vi "pulse_distribute_tester.vi"() -> ()   [LabVIEW 2021]
uses:
  <instrlib>/_niInstr/DSP/v1/Shared/Public/IQ Data.ctl
  pdw.ctl
  mode_type.ctl
  <instrlib>/_niInstr/Basic Elements/v1/FPGA/Private/Count Up U64.vi
  <instrlib>/_niInstr/Basic Elements/v1/FPGA/niInstr Basic Elements v1 FPGA.lvlib
  <instrlib>/_niInstr/DSP/v1/Shared/niInstr DSP v1 Shared.lvlib
panel:
  out "pulses read":u64=36
  out "free dds 4":bool=TRUE
  out "free dds 3":bool
  out "free dds 2":bool
  out "free dds":bool
  out "Boolean 4":bool
  out "Boolean 3":bool
  out "Boolean 2":bool
  out "Boolean":bool
  out "time":u64=655
  in  "stop":bool
  out "new pulse":bool
  out "free DDS":bool[](array[boolean])=[FALSE, FALSE, FALSE, TRUE]
  out "output cluster":T1 {"I" format="%#_6f"}
  out "get new poulse":bool=TRUE
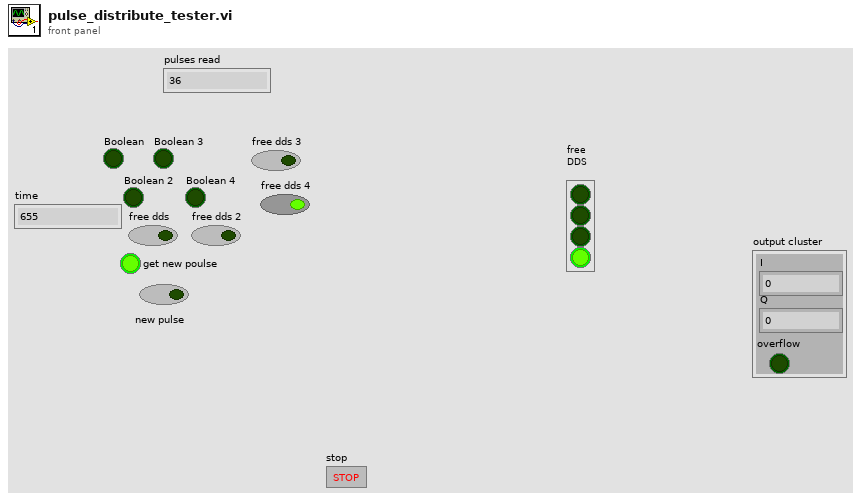
[diagram p1: front panel]
types:
  T1 = typedef "niInstr DSP v1 Shared.lvlib/IQ Data.ctl" = cluster{"I":fxp<+/-,18,1>, "Q":fxp<+/-,18,1>, "overflow":bool}
  T2 = typedef "pdw.ctl" = cluster{"PW":u32, "frequency shift":fxp<+/-,48,0>, "amp":fxp<+/-,18,1>, "mode type":T3, "mode depth":u32, "mode filter":u8, "phase shift":fxp<+/-,16,1>, "pulse shape filter":u8}
  T3 = typedef "mode_type.ctl" = enum8{"CW", "NC - CW", "NC - cw", "LFM", "BPSK", "QPSK"}
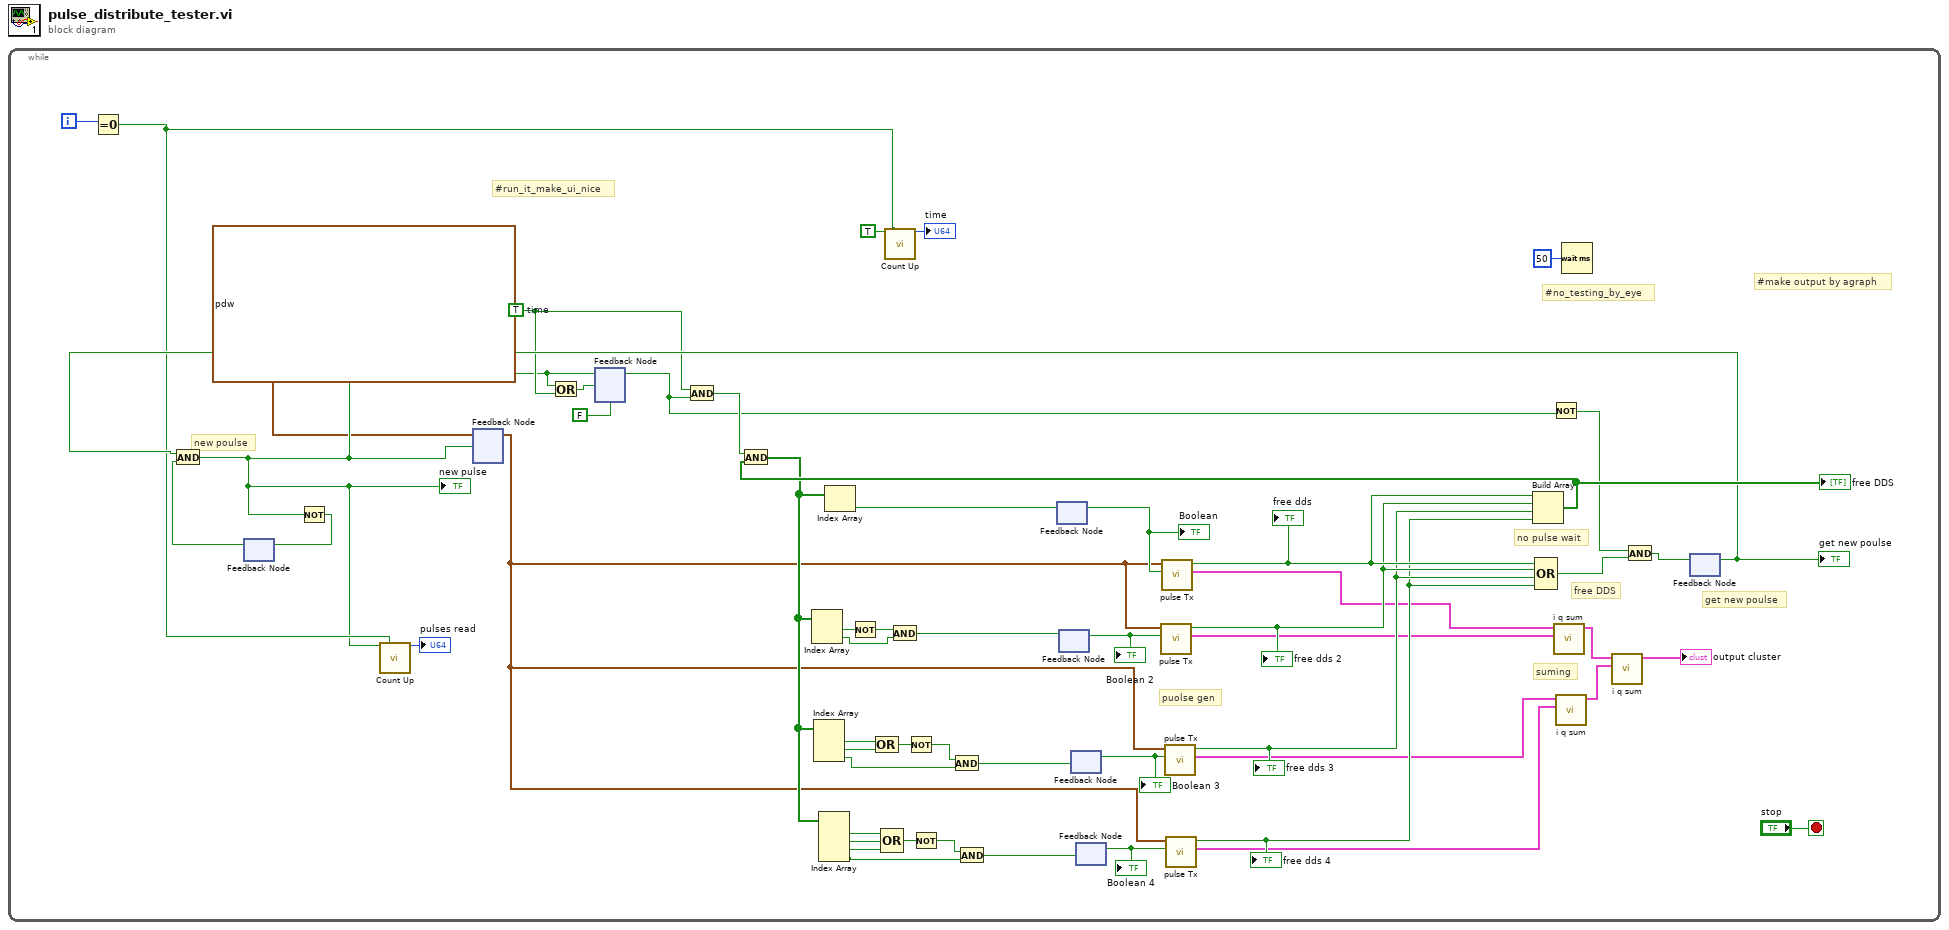
[diagram p0: block diagram]
diagram:
  n1 = while {
    i -> [w9]
    stop <- "stop" stop-if-true
    w5 = TRUE  # time
    # "#no_testing_by_eye"
    # "#make output by agraph"
    # "#run_it_make_ui_nice"
    # "new poulse"
    # "suming"
    # "puolse gen"
    # "get new poulse"
    # "no pulse wait"
    # "free DDS"
    n2 = Equal To 0?(x=w9) -> (x = 0?=w8:bool)
    n3 = feedback #1() -> (w11:bool)  [unwired: 1 in]
    n4 = feedback #2() -> (w1:T2)  [unwired: 1 in]
    n5 = feedback #3(FALSE ("Output Valid")) -> (w3:bool)
    n6 = And(x=w5, y=w3) -> (x .and. y?=w35:bool)
    n7 = call-poly <instrlib>:"Count Up.vi"("increment"=TRUE, "reset"=w8) -> ("count out"=→"time":u64)  [unwired: 13 in]
    n8 = feedback #4() -> (w23:bool)  [unwired: 1 in]
    "Boolean" <- w23
    n9 = feedback #5() -> (w46:bool)  [unwired: 1 in]
    "Boolean 2" <- w46
    n10 = feedback #6() -> (w45:bool)  [unwired: 1 in]
    "Boolean 3" <- w45
    n11 = feedback #7() -> (w43:bool)  [unwired: 1 in]
    "Boolean 4" <- w43
    n12 = call "pulse Tx.vi"("take it!"=w46, "Cluster"=w1) -> ("data out"=w29:T1, "free dds"=w55:bool)  [unwired: 5 in, 3 out]
    "free dds 2" <- w55
    n13 = call "pulse Tx.vi"("take it!"=w23, "Cluster"=w1) -> ("data out"=w30:T1, "free dds"=w56:bool)  [unwired: 5 in, 3 out]
    "free dds" <- w56
    n14 = call "pulse Tx.vi"("take it!"=w45, "Cluster"=w1) -> ("data out"=w28:T1, "free dds"=w44:bool)  [unwired: 5 in, 3 out]
    "free dds 3" <- w44
    n15 = call "pulse Tx.vi"("take it!"=w43, "Cluster"=w1) -> ("data out"=w27:T1, "free dds"=w36:bool)  [unwired: 5 in, 3 out]
    "free dds 4" <- w36
    n16 = Build Array(w56, w55, w44, w36) -> (w34:bool[])
    "free DDS" <- w34
    n17 = And(x=w35, y=w34) -> (x .and. y?=w33:bool[])
    n18 = Index Array(array=w33) -> (element #1=w54:bool, element #2=w52:bool)  [unwired: 2 in]
    n19 = Index Array(array=w33) -> (element #1=w48:bool, element #2=w49:bool, element #3=w50:bool)  [unwired: 3 in]
    n20 = Index Array(array=w33) -> (element #1=w41:bool, element #2=w40:bool, element #3=w37:bool, element #4=w38:bool)  [unwired: 4 in]
    n21 = Index Array(array=w33) -> (element=w17:bool)  [unwired: 1 in]
    n22 = Not(x=w54) -> (.not. x?=w53:bool)
    n23 = Compound Arithmetic op=OR(w48, w49) -> (w47:bool)
    n24 = Compound Arithmetic op=OR(w41, w40, w37) -> (w42:bool)
    n25 = And(x=w53, y=w52) -> (x .and. y?=w16:bool)
    n26 = Not(x=w47) -> (.not. x?=w51:bool)
    n27 = Not(x=w42) -> (.not. x?=w39:bool)
    n28 = And(x=w51, y=w50) -> (x .and. y?=w15:bool)
    n29 = And(x=w39, y=w38) -> (x .and. y?=w14:bool)
    n30 = feedback-in #4(w17) -> ()
    n31 = feedback-in #5(w16) -> ()
    n32 = feedback-in #6(w15) -> ()
    n33 = feedback-in #7(w14) -> ()
    n34 = Compound Arithmetic op=OR(w56, w55, w44, w36) -> (w31:bool)
    n35 = Not(x=w3) -> (.not. x?=w32:bool)
    n36 = call "i q sum.vi"(10:"data in"=w29, 11:"data in"=w30) -> ("output cluster"=w26:T1)  [unwired: 8 in, 1 out]
    n37 = call "i q sum.vi"(10:"data in"=w27, 11:"data in"=w28) -> ("output cluster"=w25:T1)  [unwired: 8 in, 1 out]
    n38 = Wait (ms)(milliseconds to wait=u32 50) -> ()  [unwired: 1 out]
    n39 = call "i q sum.vi"(10:"data in"=w25, 11:"data in"=w26) -> ("output cluster"=→"output cluster":T1)  [unwired: 8 in, 1 out]
    n40 = And(x=w32, y=w31) -> (x .and. y?=w18:bool)
    n41 = feedback-in #8(w18) -> ()
    n42 = feedback #8() -> (w12:bool)  [unwired: 1 in]
    "get new poulse" <- w12
    n43 = And(x=w12, y=w11) -> (x .and. y?=w4:bool)
    "new pulse" <- w4
    n44 = Not(x=w4) -> (.not. x?=w13:bool)
    n45 = feedback-in #1(w13) -> ()
    n46 = call-poly <instrlib>:"Count Up.vi"("increment"=w4, "reset"=w8) -> ("count out"=→"pulses read":u64)  [unwired: 13 in]
    n47 = feedback-in #2(T2 {"PW"=100, "frequency shift"=0.10000000000000142, "amp"=0.9999923706054688, "mode type"=enum."CW", "mode depth"=0, "mode filter"=0, "phase shift"=0.0, "pulse shape filter"=6} ("Cluster"), w4) -> ()
    n48 = Or(x=w4, y=w5) -> (x .or. y?=w6:bool)
    n49 = feedback-in #3(w4, w6) -> ()
  }
